vi "Time.vi"(8 "error in (no error)":errorcluster, 10 "Control In":T1={"I-O.lvclass"=refnum, "Gantry"=refnum, "Dispenser"="COM1"}, 11 "C4 Dispense in":refnum<class "Iterative Dispense.lvclass">) -> (0 "error out":errorcluster, 1 "Timing Data":i32[](array[numeric]), 2 "Control Out":T1={"I-O.lvclass"=refnum, "Gantry"=refnum, "Dispenser"="COM1"}, 3 "C4 Dispense out":refnum<class "Iterative Dispense.lvclass">)   [LabVIEW 2021, in "Iterative Dispense.lvclass"]
uses:
  Iterative Dispense.lvclass
  C:/Users/HEP/Documents/GitHub/Gantry/UCSB-Gantry-HEP-main/Classes/Routine/Dispense/Dispense.lvclass
  Controller/Controllers.ctl
  Controller/I-O/I-O.lvclass
  C:/Program Files (x86)/Aerotech/A3200/LabVIEW/2010/Bin/Aerotech.A3200.dll
  Program Files (x86)/Aerotech/A3200/LabVIEW/2010/Bin/Aerotech.A3200.dll
  Iterative Dispense.lvclass/Iterative Dispense.ctl
  Controller/Motion/Motion.lvclass
  Controller/Motion/A3200/A3200.lvclass
  Controller/Controller.lvclass
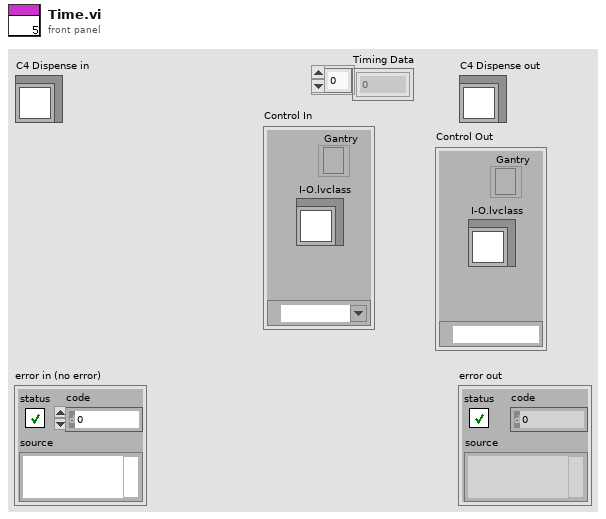
[diagram p1: front panel]
types:
  T1 = typedef "Controller.lvclass/Controllers.ctl" = cluster{"I-O.lvclass":refnum<class "I-O.lvclass">, "Gantry":refnum<k24>, "Dispenser":refnum<visa-resource-name>}
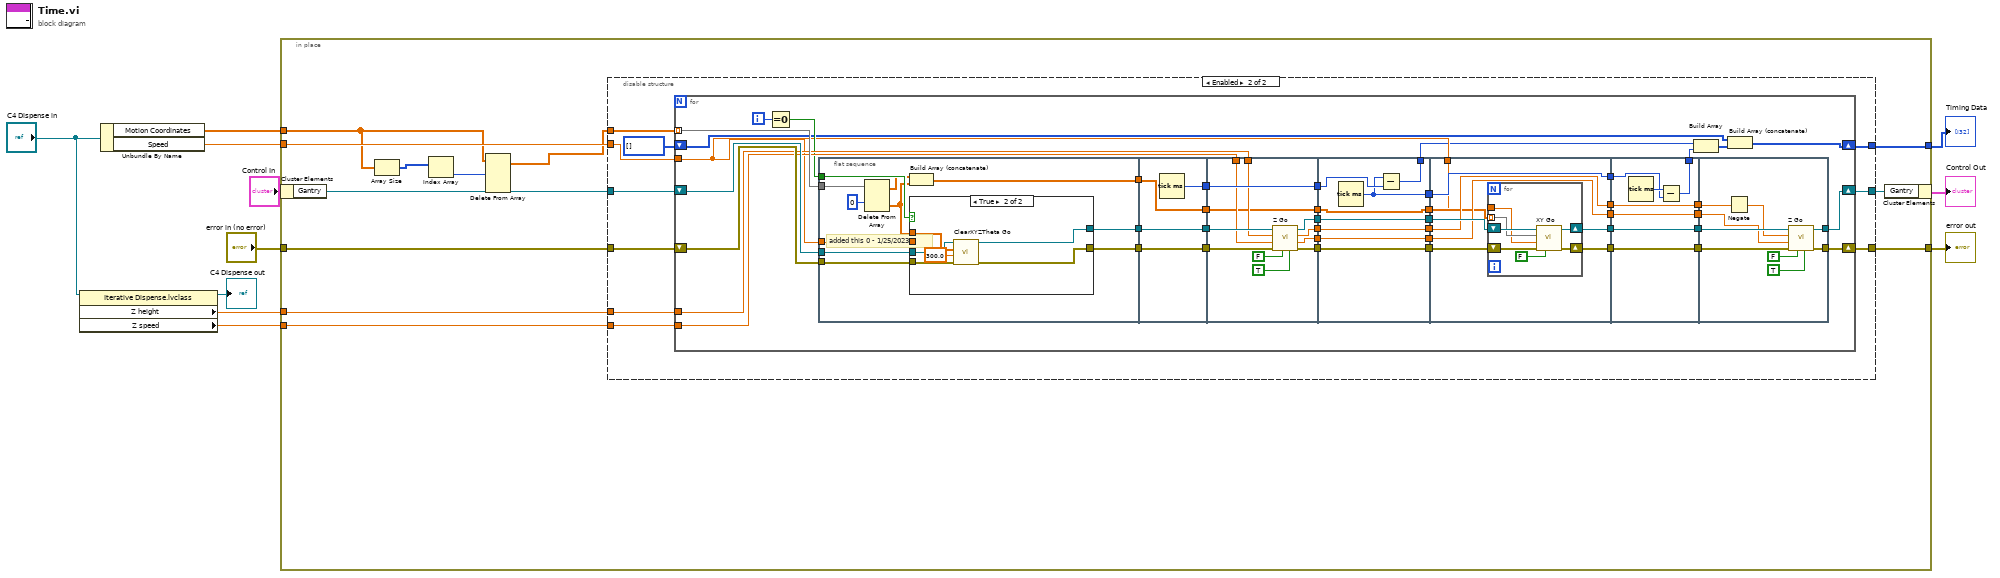
[diagram p0: block diagram]
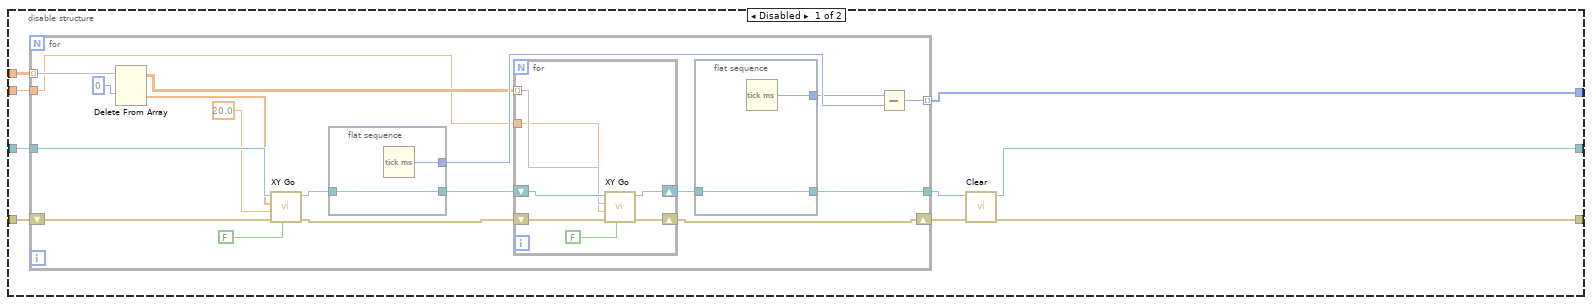
[diagram p2: hidden frame]
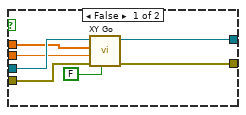
[diagram p3: hidden frame]
diagram:
  n1 = property class="Iterative Dispense.lvclass"(reference="C4 Dispense in") -> (reference out=→"C4 Dispense out":refnum<class "Iterative Dispense.lvclass">, "Z height"=w1:dbl, "Z speed"=w2:dbl)  [unwired: 1 in, 1 out]
  n2 = Unbundle By Name("C4 Dispense in") -> ("Motion Coordinates"=w11:dbl[][][], "Speed"=w7:dbl)
  n3 = in-place {
    in-place-border: w11 -> [w15]
    in-place-border: [w23] -> w10
    in-place-border: w7 -> [w22]
    in-place-border: "error in (no error)" -> [w19]
    in-place-border: [w18] -> w5
    in-place-border: w2 -> [w17]
    in-place-border: w1 -> [w16]
    n4 = in-place-cluster #1("Control In") -> ("Gantry"=w21:refnum<k24>)
    n5 = Array Size(array=w15) -> (size(s)=w14:i32[])
    n6 = Index Array(array=w14) -> (element=w13:i32)  [unwired: 1 in]
    n7 = Delete From Array(array=w15, index (dim 0)=w13) -> (array with subset deleted=w12:dbl[][][])  [unwired: 3 in, 1 out]
    n8 = disable-structure shown="Enabled" {
      disable-tunnel: w12 -> [w32 w71]
      disable-tunnel: [w31 w63] -> w23
      disable-tunnel: w22 -> [w30 w66]
      disable-tunnel: w21 -> [w29 w70]
      disable-tunnel: [w28 w65] -> w20
      disable-tunnel: w19 -> [w26 w69]
      disable-tunnel: [w24 w64] -> w18
      disable-tunnel: w17 -> [_ w68]
      disable-tunnel: w16 -> [_ w67]
      frame Disabled {
        n9 = for {
          tunnel: [w48] -> w31 mode=indexing
          tunnel: w32 -> [w45] mode=indexing
          tunnel: w30 -> [w44]
          tunnel: w29 -> [w42]
          tunnel: [w39] -> w27
          shift-right: [w34] -> w25
          shift-left: w26 -> [w36]
          n10 = Delete From Array(array=w45, index (row)=0) -> (deleted portion=w38:dbl[], array with subset deleted=w47:dbl[][])  [unwired: 2 in]
          n11 = call "XY Go.vi"("return immediately"=FALSE, "error in (no error)"=w36, "Speed"=20.0, "XY In"=w38, "Gantry In"=w42) -> ("error out"=w35:errorcluster, "Gantry Out"=w41:refnum<k24>)  [unwired: 4 in, 1 out]
          n12 = flat-sequence {
            tunnel: [w54] -> w50
            tunnel: w41 -> [w53]
            tunnel: [w53] -> w40
            frame #0 {
              n13 = Tick Count (ms)() -> (millisecond timer value=w54:u32)
            }
          }
          n14 = for {
            tunnel: w47 -> [w59] mode=indexing
            tunnel: w44 -> [w58]
            shift-right: [w60] -> w43
            shift-left: w40 -> [w61]
            shift-right: [w56] -> w34
            shift-left: w35 -> [w57]
            n15 = call "XY Go.vi"("return immediately"=FALSE, "error in (no error)"=w57, "Speed"=w58, "XY In"=w59, "Gantry In"=w61) -> ("error out"=w56:errorcluster, "Gantry Out"=w60:refnum<k24>)  [unwired: 4 in, 1 out]
          }
          n16 = flat-sequence {
            tunnel: [w52] -> w49
            tunnel: [w51] -> w39
            tunnel: w43 -> [w51]
            frame #0 {
              n17 = Tick Count (ms)() -> (millisecond timer value=w52:u32)
            }
          }
          n18 = Subtract(x=w49, y=w50) -> (x-y=w48:u32)
        }
        n19 = call "Clear.vi"("error in (no error)"=w25, "Gantry In"=w27) -> ("error out"=w24:errorcluster, "Gantry Out"=w28:refnum<k24>)  [unwired: 8 in]
      }
      frame Enabled {
        n20 = for {
          tunnel: w71 -> [w89] mode=indexing
          tunnel: w68 -> [w87]
          tunnel: w67 -> [w86]
          tunnel: w66 -> [w77]
          shift-right: [w81] -> w65
          shift-left: w70 -> [w90]
          shift-right: [w80] -> w64
          shift-left: w69 -> [w88]
          shift-right: [w72] -> w63
          shift-left: u32[] [] -> [w75]
          i -> [w79]
          n21 = Equal To 0?(x=w79) -> (x = 0?=w78:bool)
          n22 = flat-sequence {
            tunnel: [w125] -> w114
            tunnel: [w124] -> w113
            tunnel: w90 -> [w123]
            tunnel: w89 -> [w122]
            tunnel: w88 -> [w121]
            tunnel: [w116] -> w82
            tunnel: w78 -> [w120]
            tunnel: w77 -> [w119]
            tunnel: w114 -> [w141]
            tunnel: [w141] -> w112
            tunnel: [w142] -> w111
            tunnel: [w140] -> w110
            tunnel: w113 -> [w140]
            tunnel: [w139] -> w83
            tunnel: w82 -> [w139]
            tunnel: w112 -> [w154]
            tunnel: [w153] -> w109
            tunnel: w111 -> [w153]
            tunnel: [w152] -> w108
            tunnel: [w151] -> w107
            tunnel: [w150] -> w106
            tunnel: w110 -> [w149]
            tunnel: [w148] -> w105
            tunnel: w87 -> [w145]
            tunnel: w86 -> [w144]
            tunnel: [w143] -> w84
            tunnel: w83 -> [w143]
            tunnel: w109 -> [w162]
            tunnel: [w161] -> w73
            tunnel: [w160] -> w104
            tunnel: w108 -> [w160]
            tunnel: [w159] -> w103
            tunnel: [w158] -> w102
            tunnel: w107 -> [w158]
            tunnel: [w157] -> w101
            tunnel: w106 -> [w157]
            tunnel: w105 -> [w156]
            tunnel: [w156] -> w100
            tunnel: [w155] -> w85
            tunnel: w84 -> [w155]
            tunnel: w104 -> [w171]
            tunnel: [w170] -> w99
            tunnel: w103 -> [w170]
            tunnel: [w169] -> w98
            tunnel: [w168] -> w97
            tunnel: w102 -> [w168]
            tunnel: [w167] -> w96
            tunnel: w101 -> [w167]
            tunnel: w100 -> [w166]
            tunnel: [w165] -> w95
            tunnel: w85 -> [w164]
            tunnel: w77 -> [w163]
            tunnel: w99 -> [w184]
            tunnel: [w183] -> w94
            tunnel: w98 -> [w183]
            tunnel: [w182] -> w93
            tunnel: w97 -> [w182]
            tunnel: [w181] -> w92
            tunnel: w96 -> [w181]
            tunnel: [w180] -> w91
            tunnel: w95 -> [w180]
            tunnel: [w179] -> w74
            tunnel: w94 -> [w194]
            tunnel: w93 -> [w193]
            tunnel: w92 -> [w191]
            tunnel: [w190] -> w81
            tunnel: w91 -> [w189]
            tunnel: [w188] -> w80
            frame #0 {
              # "added this 0 - 1/25/2023"
              n23 = Delete From Array "Delete From Array"(array=w122, index (row)=0) -> (deleted portion=w117:dbl[], array with subset deleted=w118:dbl[][])  [unwired: 2 in]
              n24 = Build Array (concatenate)(w118, w117) -> (w116:dbl[][])
              n25 = case shown="True" w120 {
                tunnel: [w132 w138] -> w125
                tunnel: [w131 w137] -> w124
                tunnel: w123 -> [w128 w136]
                tunnel: w117 -> [w127 w135]
                tunnel: w121 -> [w129 w134]
                tunnel: w119 -> [w126 _]
                frame False {
                  n26 = call "XY Go.vi"("return immediately"=FALSE, "error in (no error)"=w129, "Speed"=w126, "XY In"=w127, "Gantry In"=w128) -> ("error out"=w131:errorcluster, "Gantry Out"=w132:refnum<k24>)  [unwired: 4 in, 1 out]
                }
                frame True {
                  n27 = call "ClearXYZTheta Go.vi"("error in (no error)"=w134, "Speed"=300.0, "XYZTheta In"=w135, "Gantry In"=w136) -> ("error out"=w137:errorcluster, "Gantry Out"=w138:refnum<k24>)  [unwired: 5 in, 1 out]
                }
              }
            }
            frame #1 {
              n28 = Tick Count (ms)() -> (millisecond timer value=w142:u32)
            }
            frame #2 {
              n29 = call "Z Go.vi"("Increment"=TRUE, "Return Immediately"=FALSE, "error in (no error)"=w149, "Speed In"=w145, "Position In"=w144, "Gantry In"=w154) -> ("error out"=w148:errorcluster, "Speed Out"=w150:dbl, "Position Out"=w151:dbl, "Gantry Out"=w152:refnum<k24>)  [unwired: 2 in]
            }
            frame #3 {
              n30 = Tick Count (ms)() -> (millisecond timer value=w159:u32)
              n31 = Subtract(x=w159, y=w162) -> (x-y=w161:u32)
            }
            frame #4 {
              n32 = for {
                shift-right: [w177] -> w169
                shift-left: w171 -> [w178]
                shift-right: [w175] -> w165
                shift-left: w166 -> [w176]
                tunnel: w164 -> [w173] mode=indexing
                tunnel: w163 -> [w172]
                n33 = call "XY Go.vi"("return immediately"=FALSE, "error in (no error)"=w176, "Speed"=w172, "XY In"=w173, "Gantry In"=w178) -> ("error out"=w175:errorcluster, "Gantry Out"=w177:refnum<k24>)  [unwired: 4 in, 1 out]
              }
            }
            frame #5 {
              n34 = Tick Count (ms)() -> (millisecond timer value=w185:u32)
              n35 = Subtract(x=w185, y=w184) -> (x-y=w179:u32)
            }
            frame #6 {
              n36 = Negate(x=w193) -> (-x=w192:dbl)
              n37 = call "Z Go.vi"("Increment"=TRUE, "Return Immediately"=FALSE, "error in (no error)"=w189, "Speed In"=w191, "Position In"=w192, "Gantry In"=w194) -> ("error out"=w188:errorcluster, "Gantry Out"=w190:refnum<k24>)  [unwired: 2 in, 2 out]
            }
          }
          n38 = Build Array(w73, w74) -> (w76:u32[])
          n39 = Build Array (concatenate)(w75, w76) -> (w72:u32[])
        }
      }
    }
    n40 = in-place-cluster #1("Gantry"=w20) -> (→"Control Out":T1)
  }
  "error out" <- w5
  "Timing Data" <- w10
